vi "Config Process.vi"(8 "error in (no error)":errorcluster, 11 "Variables":T1) -> (0 "error out":errorcluster, 3 "Variables":T1)   [LabVIEW 2017]
doc: "Realized configuration process for reading data from DB"
uses:
  support/Controls/Shared Variables.ctl
  Controls/ConfigData.ctl
  Elevator/Controls/Elevator Overhead.ctl
  Elevator/Controls/Elevator States.ctl
  Elevator/Controls/Elevator Location.ctl
  Elevator/Controls/Elevator Command Event.ctl
  Elevator/Controls/Elevator Commands.ctl
  Error Handler/Controls/Error EventData.ctl
  Error Handler/Controls/Error Type.ctl
  support/Controls/User Events.ctl
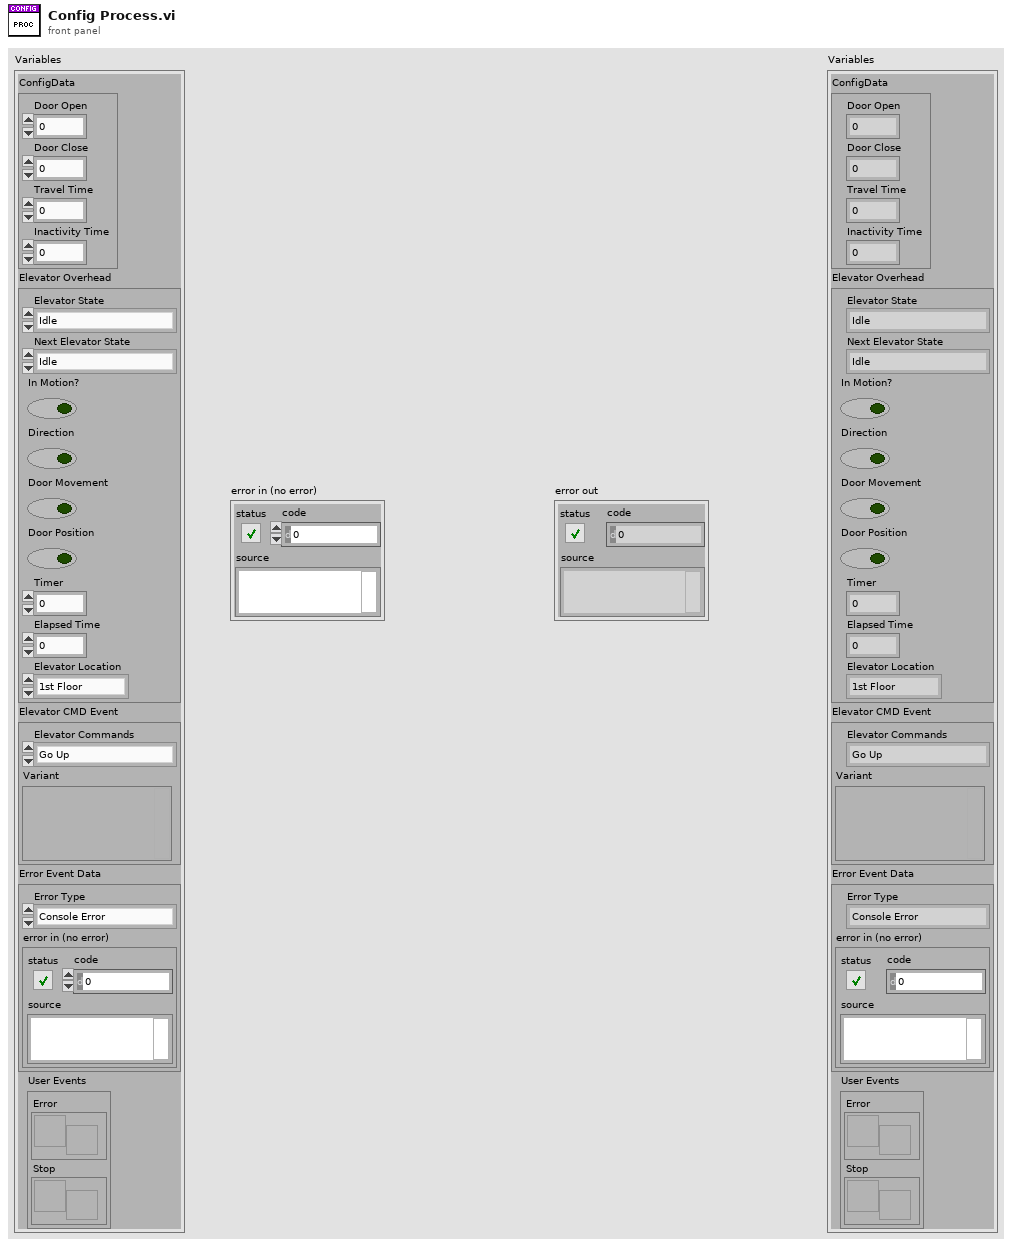
[diagram p1: front panel]
types:
  T1 = typedef "Shared Variables.ctl" = cluster{"ConfigData":T2, "Elevator Overhead":T3, "Elevator CMD Event":T6, "Error Event Data":T8, "User Events":T10}
  T2 = typedef "ConfigData.ctl" = cluster{"Door Open":dbl, "Door Close":dbl, "Travel Time":dbl, "Inactivity Time":dbl}
  T3 = typedef "Elevator Overhead.ctl" = cluster{"Elevator State":T4, "Next Elevator State":T4, "In Motion?":bool, "Direction":bool, "Door Movement":bool, "Door Position":bool, "Timer":dbl, "Elapsed Time":dbl, "Elevator Location":T5}
  T4 = typedef "Elevator States.ctl" = enum16{"Idle", "Init", "Open Doors", "Close Doors", "Start Move", "Move", "Finish Move", "Analysis", "Emergency"}
  T5 = typedef "Elevator Location.ctl" = enum16{"1st Floor", "2nd Floor", "3rd Floor", "4th Floor"}
  T6 = typedef "Elevator Command Event.ctl" = cluster{"Elevator Commands":T7, "Variant":variant}
  T7 = typedef "Elevator Commands.ctl" = enum16{"Go Up", "Go Down", "Go to Floor", "Emergency", "Open Doors", "Close Doors"}
  T8 = typedef "Error EventData.ctl" = cluster{"Error Type":T9, "error in (no error)":errorcluster}
  T9 = typedef "Error Type.ctl" = enum16{"Console Error", "Sensor Interface IO Error", "Process Step Error"}
  T10 = typedef "User Events.ctl" = cluster{"Error":refnum<user-event>, "Stop":refnum<user-event>}
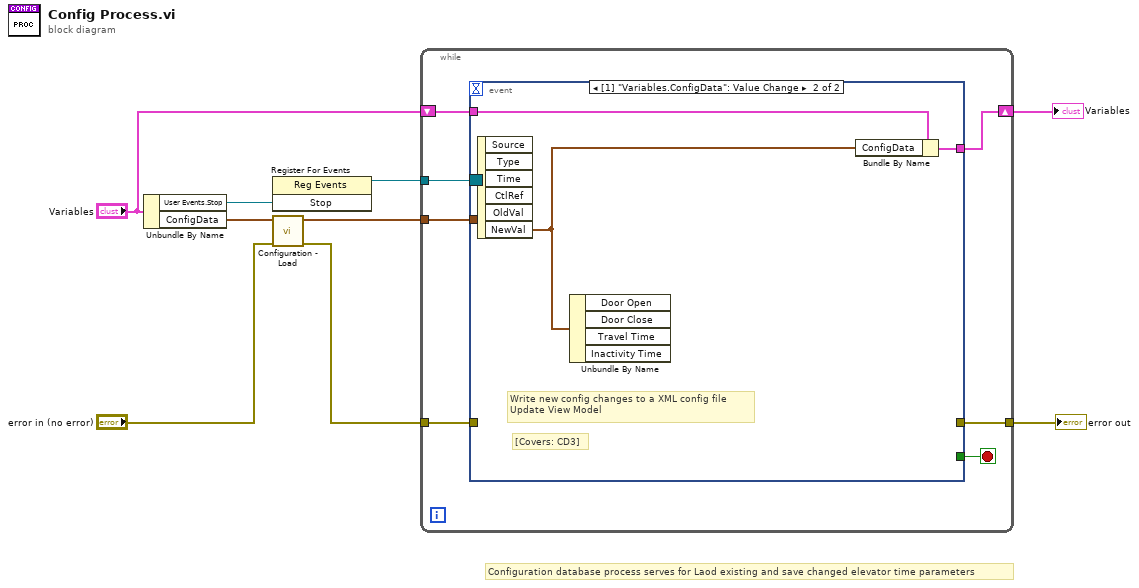
[diagram p0: block diagram]
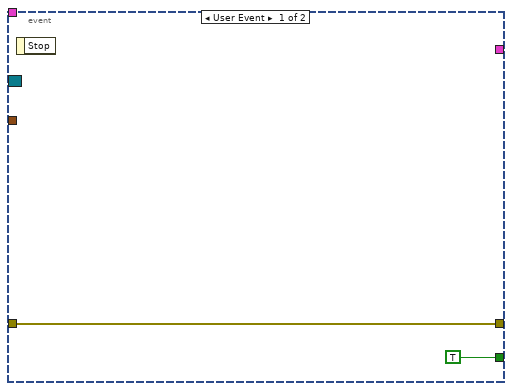
[diagram p2: hidden frame]
diagram:
  # "Configuration database process serves for Laod existing and save changed elevator time parameters"
  n1 = Unbundle By Name("Variables") -> ("User Events.Stop"=w9:refnum<user-event>, "ConfigData"=w6:T2)
  n2 = register-events(w9) -> (reference out=w8:refnum<event-registration>)  [unwired: 2 in, 1 out]
  n3 = call "Configuration - Load.vi"("error in (no error)"="error in (no error)", "Configuration Data"=w6) -> ("error out"=w3:errorcluster, "Configuration Data"=w5:T2)  [unwired: 8 in]
  n4 = while {
    tunnel: w8 -> [w16]
    tunnel: w3 -> [w14]
    tunnel: [w13] -> w7
    tunnel: w5 -> [w12]
    shift-right: [w10] -> w1
    shift-left: "Variables" -> [w11]
    stop <- w15 stop-if-true
    n5 = event shown="[1] \"Variables.ConfigData\": Value Change" {
      selector: w16 -> [_ _]
      dyn-events: _ -> [_ _]
      timeout: _ -> [_ _]
      tunnel: [TRUE _] -> w15
      tunnel: w14 -> [w17 _]
      tunnel: [w17 _] -> w13
      tunnel: w12 -> [_ _]
      tunnel: w11 -> [_ w21]
      tunnel: [_ w19] -> w10
      event User Event {
        n6 = event-data() -> ()  [unwired: 1 in, 1 out]
      }
      event Value Change {
        # "[Covers: CD3]"
        # "Write new config changes to a XML config file\nUpdate View Model"
        n7 = event-data() -> ("NewVal"=w20:T2)  [unwired: 1 in, 5 out]
        n8 = Unbundle By Name(w20) -> ()  [unwired: 4 out]
        n9 = Bundle By Name(cluster=w21, "ConfigData"=w20) -> (w19:T1)
      }
    }
  }
  "error out" <- w7
  "Variables" <- w1
